vi "Password Popup.vi"(8 "error in":errorcluster) -> (0 "error out":errorcluster, 3 "Password out":string)   [LabVIEW 2018]
uses:
  <vilib>/event_ctls.llb/eventvkey.ctl
panel:
  in  "OK":bool
  in  "Password":string
  # "password"
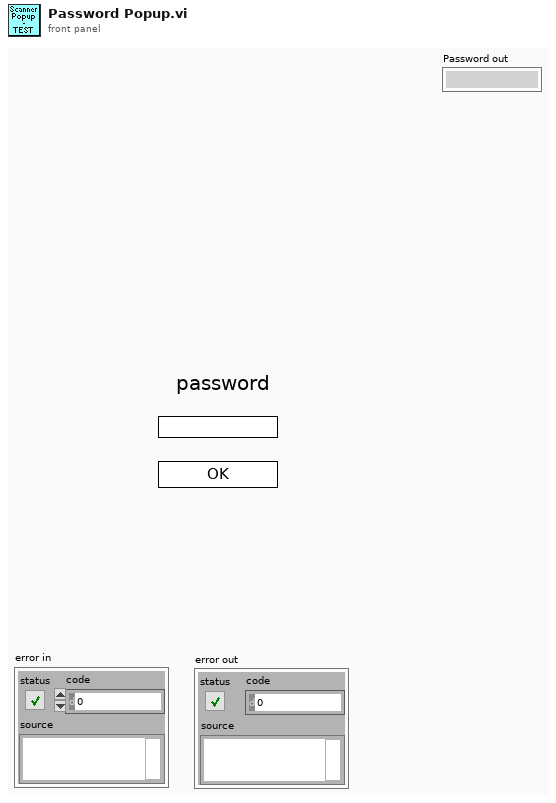
[diagram p1: front panel]
types:
  T1 = typedef "eventvkey.ctl" = enum16{"ASCII", "Enter", "Return", "Shift", "Ctrl", "Alt", "Cmd", "Opt", "Caps", "NumLock", "Clear", "Break", "Up", "Down", "Left", "Right", "Insert", "Delete", "Home", "End", "PageUp", "PageDown", "Escape", "Help", "Pause", "ScrollLock", "F1", "F2", "F3", "F4", "F5", "F6", "F7", "F8", "F9", "F10", "F11", "F12", "F13", "F14", "F15", "F16", "F17", "F18", "F19", "F20", "F21", "F22", "F23", "F24", "Play", "VolumeUp", "VolumeDown", "Mute", "Two Byte Char"}
  T2 = enum8{"Enabled", "Disabled", "Disabled and Grayed Out"}
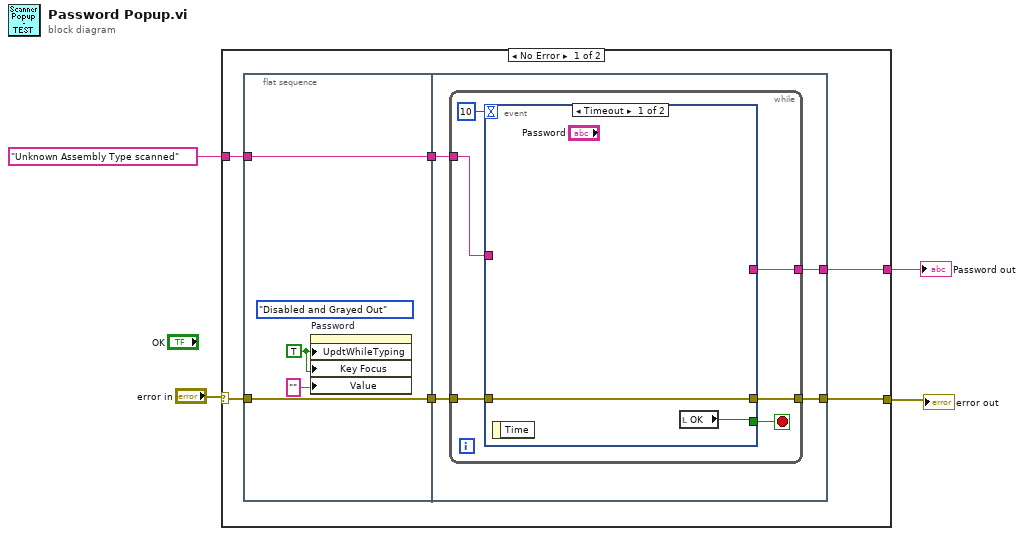
[diagram p0: block diagram]
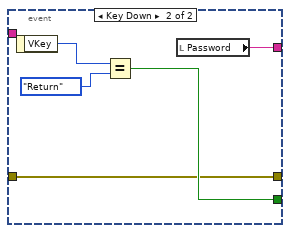
[diagram p2: hidden frame]
diagram:
  n1 = case shown="No Error" "error in" {
    selector: "error in" -> [w9 w32]
    tunnel: [w8 w32] -> w3
    tunnel: [w7 _] -> w2
    tunnel: "Unknown Assembly Type scanned" ("Error") -> [w5 _]
    frame No Error {
      n2 = flat-sequence {
        tunnel: [w14] -> w10
        tunnel: w9 -> [w14]
        tunnel: [w11] -> w6
        tunnel: w5 -> [w11]
        tunnel: w10 -> [w16]
        tunnel: [w17] -> w8
        tunnel: [w18] -> w7
        tunnel: w6 -> [w15]
        frame #0 {
          w13 = TRUE ("Update While Typing?")
          (unwired) T2."Disabled and Grayed Out" ("Disabled")
          n3 = property on="Password" class="Str"("UpdtWhileTyping"=w13, "Key Focus"=w13, "Value"="" ("Module SN")) -> ()  [unwired: 2 in, 2 out]
        }
        frame #1 {
          n4 = while {
            tunnel: [w24] -> w18
            tunnel: [w20] -> w17
            tunnel: w16 -> [w23]
            tunnel: w15 -> [w19]
            stop <- w21 stop-if-true
            n5 = event shown="[0] Timeout" {
              selector: _ -> [_ _]
              dyn-events: _ -> [_ _]
              timeout: 10 -> [_ _]
              tunnel: [_ w27] -> w24
              tunnel: w23 -> [w26 w28]
              tunnel: [w25 w29] -> w21
              tunnel: [w26 w28] -> w20
              tunnel: w19 -> [_ _]
              event Timeout {
                n6 = event-data() -> ()  [unwired: 1 in, 1 out]
                n7 = local read "OK"() -> (w25:bool)
              }
              event Key Down {
                n8 = event-data() -> ("VKey"=w31:T1)  [unwired: 1 in]
                n9 = Equal?(x=w31, y=eventvkey."Return" ("VKey")) -> (x = y?=w29:bool)
                n10 = local read "Password"() -> (w27:string)
              }
            }
          }
        }
      }
    }
    frame Error {
    }
  }
  "error out" <- w3
  "Password out" <- w2
